vi "hit_detection.vi"(7 "mod":T1, 8 "error in":errorcluster, 9 "hammerIndex":i32, 10 "config":T2={"rate"=1652.0, "duration"=1.0, "thr"=100.0, "preTrigger"=100.0, "cutoff"=-3.0, "Filtro"=enum."Desativado", "highPass"=1000.0, "lowPass"=1000.0, "updateTime"=50.0} {"updateTime" format="%#_g ms"; "lowPass" format="%#_g Hz"; "highPass" format="%#_g Hz"; "cutoff" format="%#_g dB"; "preTrigger" format="%#_g ms"; "thr" format="%#_g N"; "duration" format="%#_g s"; "rate" min=1652.0 max=51200.0 format="%#_g Hz"}, 11 "data":dbl[][](array[numeric])) -> (0 "error out":errorcluster)   [LabVIEW 2016]
uses:
  MainFGV/Settings/Advanced/AdvancedConfig.ctl
  processing_mods.ctl
  hit_detection_mods.ctl
  hold_data_mods.ctl
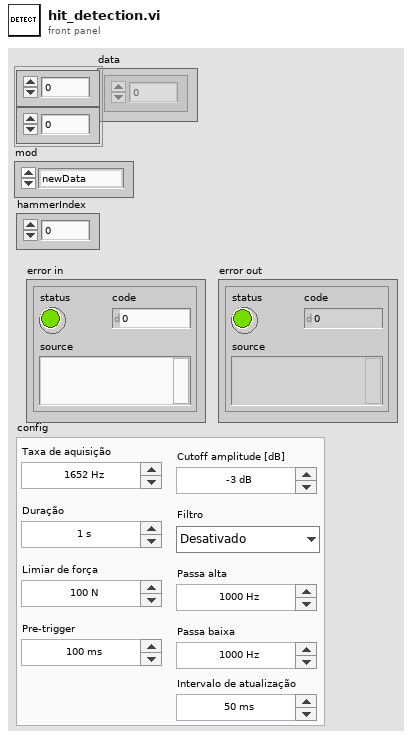
[diagram p1: front panel]
types:
  T1 = typedef "processing_mods.ctl" = enum16{"newData", "SetConfig", "setHammer"}
  T2 = typedef "AdvancedConfig.ctl" = cluster{"rate":dbl, "duration":dbl, "thr":dbl, "preTrigger":dbl, "cutoff":dbl, "Filtro":enum16{"Desativado", "Passa banda", "Passa alta", "Passa baixa"}, "highPass":dbl, "lowPass":dbl, "updateTime":dbl}
  T3 = typedef "hold_data_mods.ctl" = enum16{"setTimes", "HoldPreTrigger", "HoldData"}
  T4 = typedef "hit_detection_mods.ctl" = enum16{"wait", "acumulate", "process"}
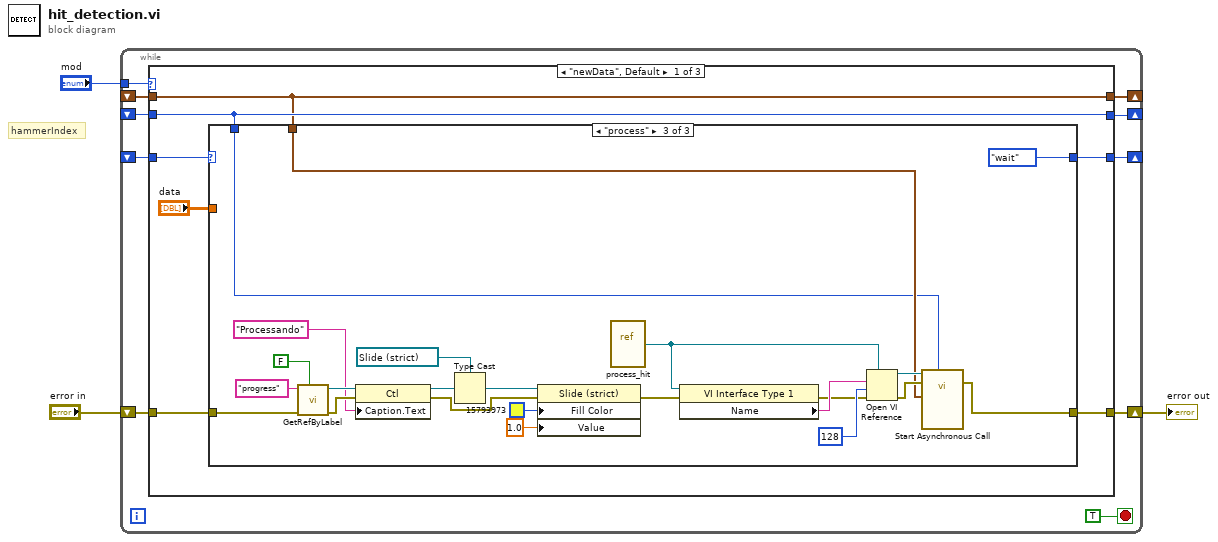
[diagram p0: block diagram]
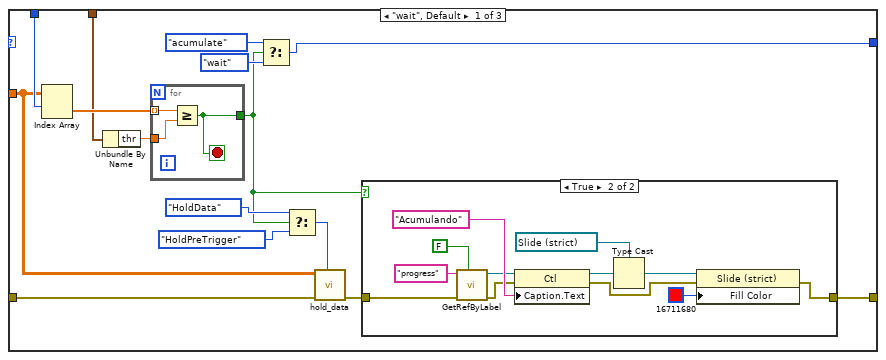
[diagram p2: hidden frame]
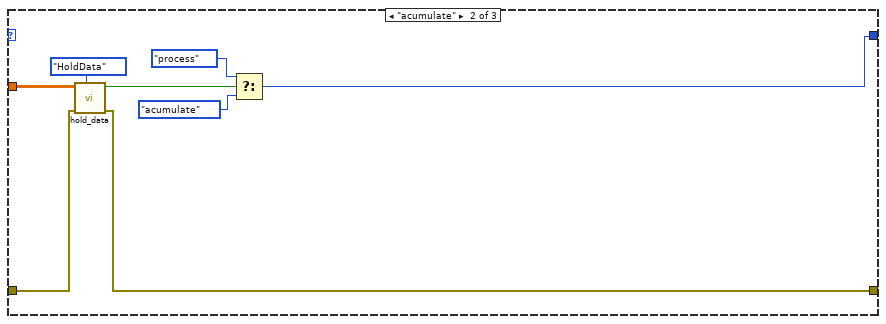
[diagram p4: hidden frame]
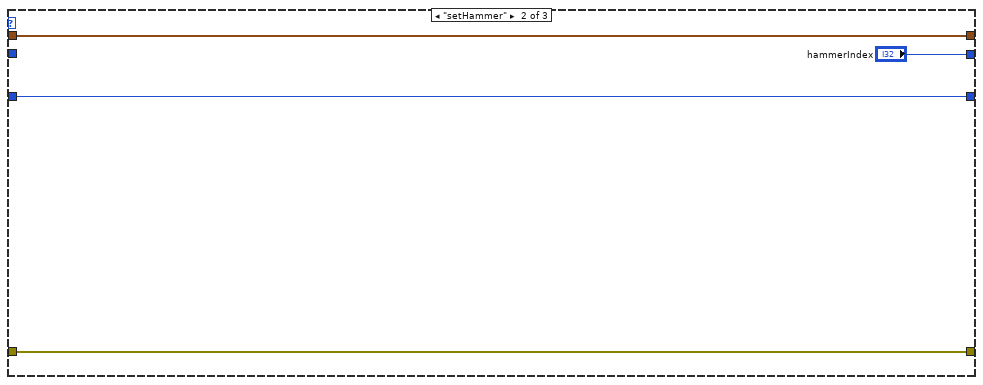
[diagram p5: hidden frame]
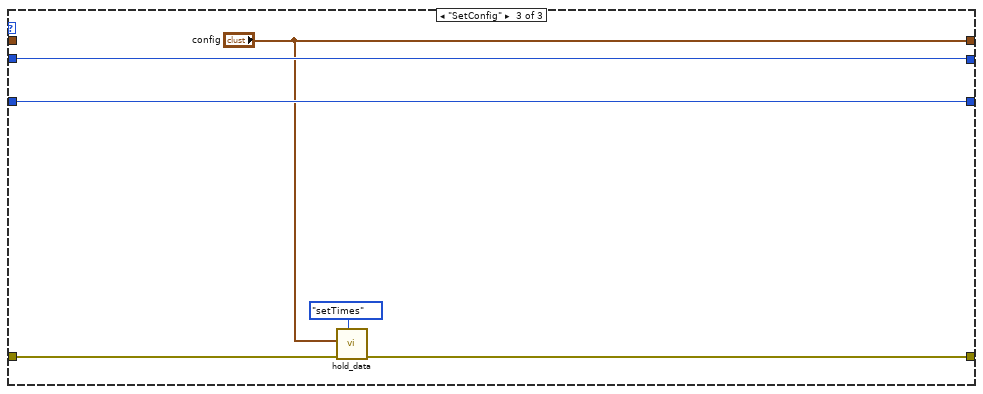
[diagram p6: hidden frame]
diagram:
  # "hammerIndex"
  n1 = while {
    tunnel: "mod" -> [w13]
    shift-right: [w11] -> _
    shift-left: _ -> [w10]
    shift-right: [w9] -> _
    shift-left: _ -> [w8]
    shift-right: [w6] -> _
    shift-left: _ -> [w7]
    shift-right: [w4] -> w1
    shift-left: "error in" -> [w5]
    stop <- TRUE stop-if-true
    n2 = case shown="\"newData\", Default" w13 {
      tunnel: [w17 w85 "config"] -> w11
      tunnel: w10 -> [w17 w85 _]
      tunnel: [w18 "hammerIndex" w92] -> w9
      tunnel: w8 -> [w18 _ w92]
      tunnel: w7 -> [w20 w84 w91]
      tunnel: [w16 w84 w91] -> w6
      tunnel: w5 -> [w15 w83 w89]
      tunnel: [w14 w83 w87] -> w4
      frame "newData", Default {
        n3 = case shown="\"process\"" w20 {
          tunnel: "data" -> [w25 w59 _]
          tunnel: w18 -> [w35 _ w60]
          tunnel: w17 -> [w33 _ w62]
          tunnel: [w29 w52 hit_detection_mods."wait"] -> w16
          tunnel: w15 -> [w27 w57 w77]
          tunnel: [w28 w56 w63] -> w14
          frame "wait", Default {
            n4 = Index Array(array=w25, index (row)=w35) -> (element=w34:dbl[])  [unwired: 1 in]
            n5 = Unbundle By Name(w33) -> ("thr"=w32:dbl)
            n6 = for {
              tunnel: w34 -> [w51] mode=indexing
              tunnel: w32 -> [w50]
              tunnel: [w49] -> w21
              stop <- w49 stop-if-true
              n7 = Greater Or Equal?(x=w51, y=w50) -> (x >= y?=w49:bool)
            }
            n8 = Select(t=hit_detection_mods."acumulate", s=w21, f=hit_detection_mods."wait") -> (s? t:f=w29:T4)
            n9 = Select(t=hold_data_mods."HoldData" ("holda_data_mod"), s=w21, f=hold_data_mods."HoldPreTrigger" ("holda_data_mod")) -> (s? t:f=w22:T3)
            n10 = call "hold_data.vi"("holda_data_mod"=w22, "Error In"=w27, "data"=w25) -> ("Error Out"=w26:errorcluster)  [unwired: 7 in, 1 out]
            n11 = case shown="True" w21 {
              tunnel: w26 -> [w36 w39]
              tunnel: [w36 w38] -> w28
              frame False {
              }
              frame True {
                n12 = call "GetRefByLabel.vi"("InsideTab"=FALSE, "error in"=w39, "Label"="progress") -> ("error out"=w41:errorcluster, "Ctl Refnum"=w42:refnum<vi>)  [unwired: 6 in, 1 out]
                n13 = property class="Ctl"(reference=w42, error in=w41, "Caption.Text"="Acumulando") -> (reference out=w45:refnum<vi>, error out=w47:errorcluster)
                n14 = Type Cast(type=refnum<vi> refnum ("progress"), x=w45) -> (*(type *) &x=w46:refnum<vi>)
                n15 = property class="Slide (strict)"(reference=w46, error in=w47, "Fill Color"=u32 16711680) -> (error out=w38:errorcluster)  [unwired: 1 out]
              }
            }
          }
          frame "acumulate" {
            n16 = call "hold_data.vi"("holda_data_mod"=hold_data_mods."HoldData", "Error In"=w57, "data"=w59) -> ("Error Out"=w56:errorcluster, "finished"=w55:bool)  [unwired: 7 in]
            n17 = Select(t=hit_detection_mods."process", s=w55, f=hit_detection_mods."acumulate") -> (s? t:f=w52:T4)
          }
          frame "process" {
            n18 = call "GetRefByLabel.vi"("InsideTab"=FALSE, "error in"=w77, "Label"="progress") -> ("error out"=w80:errorcluster, "Ctl Refnum"=w79:refnum<vi>)  [unwired: 6 in, 1 out]
            n19 = property class="Ctl"(reference=w79, error in=w80, "Caption.Text"="Processando") -> (reference out=w75:refnum<vi>, error out=w73:errorcluster)
            n20 = Type Cast(type=refnum<vi> refnum ("progress"), x=w75) -> (*(type *) &x=w74:refnum<vi>)
            n21 = property class="Slide (strict)"(reference=w74, error in=w73, "Fill Color"=u32 15793973, "Value"=1.0) -> (error out=w64:errorcluster)  [unwired: 1 out]
            n22 = vi-ref "process_hit.vi"() -> (w69:refnum<vi>)
            n23 = property class="VI Interface Type 1"(reference=w69, error in=w64) -> (error out=w67:errorcluster, "Name"=w68:string)  [unwired: 1 out]
            n24 = Open VI Reference(type specifier VI Refnum (for type only)=w69, vi path=w68, options=128, error in (no error)=w67) -> (vi reference=w66:refnum<vi>, error out=w65:errorcluster)  [unwired: 2 in]
            n25 = call-by-ref "Start Asynchronous Call"(reference=w66, error in=w65, "hammerIndex"=w60, "config"=w62) -> (error out=w63:errorcluster)  [unwired: 10 in, 1 out]
          }
        }
      }
      frame "setHammer" {
      }
      frame "SetConfig" {
        n26 = call "hold_data.vi"("holda_data_mod"=hold_data_mods."setTimes", "Error In"=w89, "config"="config") -> ("Error Out"=w87:errorcluster)  [unwired: 7 in, 1 out]
      }
    }
  }
  "error out" <- w1
